vi "8Q_backtrace.vi"(10 "Q_Num":i32=8, 11 "BT_bfr":i32[](array[numeric])=[4, 2]) -> (0 "<0_stop":bool, 2 "next_start":i32, 3 "BT_result":i32[](array[numeric]))   [LabVIEW 2012]
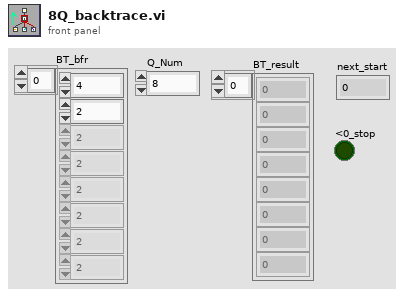
[diagram p1: front panel]
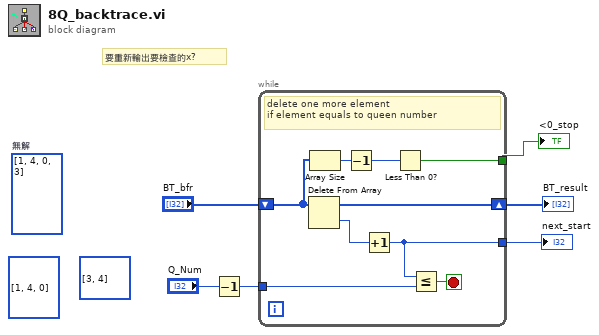
[diagram p0: block diagram]
diagram:
  (unwired) i32[] [1, 4, 0]
  (unwired) i32[] [3, 4]
  (unwired) i32[] [1, 4, 0, 3]  # 無解
  # "要重新輸出要檢查的x?"
  n1 = Decrement(x="Q_Num") -> (x-1=w1:i32)
  n2 = while {
    tunnel: [w13] -> w6
    tunnel: [w10] -> w5
    tunnel: w1 -> [w9]
    shift-right: [w8] -> w4
    shift-left: "BT_bfr" -> [w7]
    stop <- w11 stop-if-true
    # "delete one more element\nif element equals to queen number"
    n3 = Delete From Array(array=w7) -> (deleted portion=w12:i32, array with subset deleted=w8:i32[])  [unwired: 2 in]
    n4 = Array Size(array=w7) -> (size(s)=w15:i32)
    n5 = Decrement(x=w15) -> (x-1=w14:i32)
    n6 = Increment(x=w12) -> (x+1=w10:i32)
    n7 = Less Than 0?(x=w14) -> (x < 0?=w13:bool)
    n8 = Less Or Equal?(x=w10, y=w9) -> (x <= y?=w11:bool)
  }
  "BT_result" <- w4
  "next_start" <- w5
  "<0_stop" <- w6
